vi "IntegrationNtimes.vi"(0 ".NET Refnum in":refnum<k24>, 1 "Port in":string, 2 "Array in":dbl[][](array[numeric]), 3 "ComError in":bool, 4 "tEnd":dbl, 5 "Burst # (M)":u32, 6 "error in":errorcluster, 7 "error in (no error)":errorcluster, 8 "VISA Refnum in":refnum<visa-resource-name>, 9 "Restart data point":bool, 10 "Array 2":i32[](array[numeric]), 11 "# of averages (N)":i64, 12 "Array 4":dbl[][](array[numeric]), 14 "Choose experiment":T1(ring), 16 "tEndCurrent":dbl) -> (17 "Numeric":i32, 18 "VISA resource name out":refnum<visa-resource-name>, 19 "ComError out 2":bool, 20 ".NET Refnum out":refnum<k24>, 21 "Numeric 2":dbl, 22 "Array":dbl[][](array[numeric]), 23 "Array out 2":dbl[][](array[numeric]), 24 "Array 3":dbl[][](array[numeric]), 25 "error out 3":errorcluster, 26 "Port out 2":string, 27 "error out":errorcluster)   [LabVIEW 2023]
uses:
  <vilib>/ULx/ULx_LV.dll
  <vilib>/ULx/Read.llb/ULx Read (Counter 1D U32 NChan 1Samp).vi
  <instrlib>/Quantum Composers 9000 Series/Quantum Composers 9000 Series.lvlib
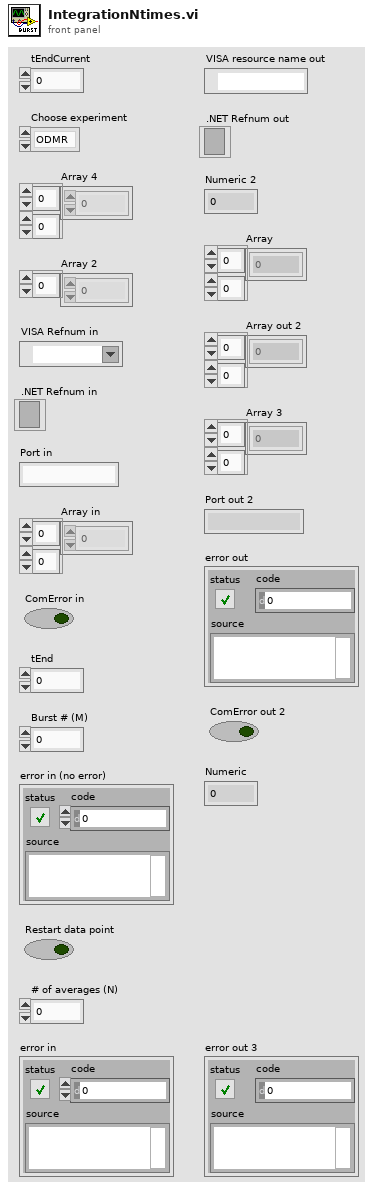
[diagram p1: front panel]
types:
  T1 = enum32{"ODMR", "Rabi", "Fidelity", "T1 Measurement"}
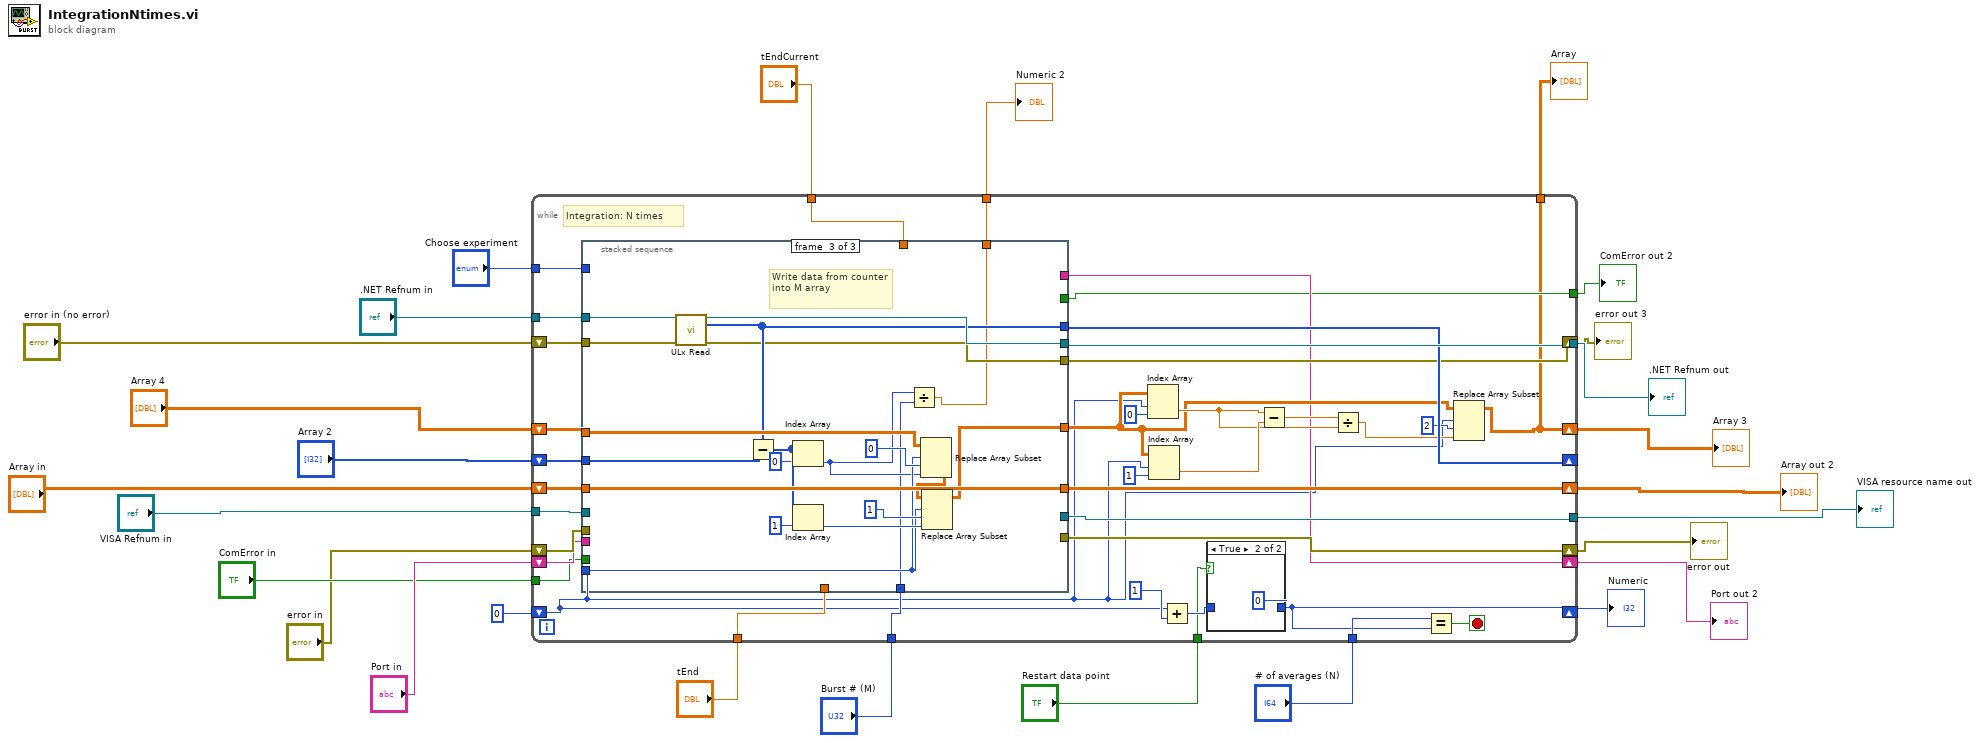
[diagram p0: block diagram]
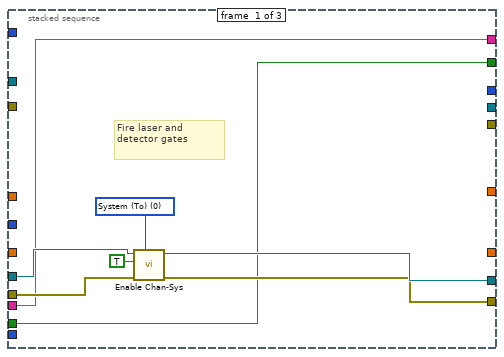
[diagram p2: hidden frame]
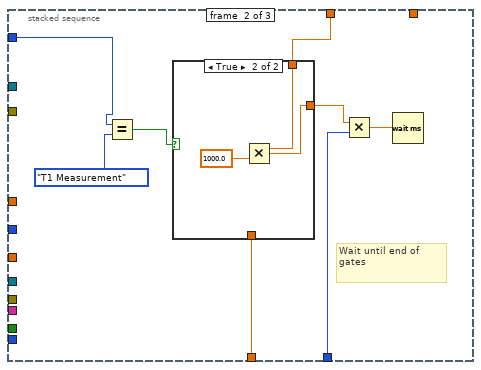
[diagram p3: hidden frame]
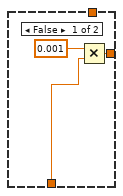
[diagram p4: hidden frame]
diagram:
  n1 = while {
    tunnel: [w65] -> w3
    tunnel: ".NET Refnum in" -> [w64]
    shift-right: [w62] -> w10
    shift-left: "Array in" -> [w61]
    shift-right: [w30] -> w7
    shift-left: "Array 4" -> [w60]
    shift-right: [w57] -> _
    shift-left: "Array 2" -> [w51]
    tunnel: [w43] -> w8
    shift-right: [w52] -> w1
    shift-left: "error in (no error)" -> [w63]
    shift-right: [w44] -> w11
    shift-left: "error in" -> [w53]
    tunnel: "VISA Refnum in" -> [w42]
    shift-right: [w40] -> w14
    shift-left: "Port in" -> [w41]
    tunnel: "ComError in" -> [w39]
    tunnel: [w38] -> w13
    tunnel: "tEndCurrent" -> [w37]
    tunnel: "Burst # (M)" -> [w36]
    tunnel: "tEnd" -> [w35]
    tunnel: "Choose experiment" -> [w34]
    tunnel: "# of averages (N)" -> [w33]
    tunnel: "Restart data point" -> [w32]
    tunnel: [w31] -> w25
    tunnel: [w30] -> w26
    shift-right: [w29] -> w27
    shift-left: 0 -> [w28]
    stop <- w54 stop-if-true
    # "Integration: N times"
    n2 = stacked-sequence {
      tunnel: w53 -> [w69 _ _]
      tunnel: w61 -> [_ _ w106]
      tunnel: [w71 _ _] -> w43
      tunnel: [_ _ w106] -> w62
      tunnel: [w70 _ _] -> w44
      tunnel: w64 -> [_ _ w104]
      tunnel: [_ _ w91] -> w52
      tunnel: [_ _ w107] -> w65
      tunnel: w63 -> [_ _ w105]
      tunnel: w28 -> [_ _ w93]
      tunnel: w60 -> [_ _ w98]
      tunnel: [_ _ w97] -> w47
      tunnel: w51 -> [_ _ w95]
      tunnel: [_ _ w96] -> w57
      tunnel: w42 -> [w68 _ _]
      tunnel: w41 -> [w67 _ _]
      tunnel: [w67 _ _] -> w40
      tunnel: w39 -> [w66 _ _]
      tunnel: [w66 _ _] -> w38
      tunnel: w37 -> [_ w77 _]
      tunnel: w36 -> [_ w76 w89]
      tunnel: w35 -> [_ w75 _]
      tunnel: w34 -> [_ w74 _]
      tunnel: [_ _ w88] -> w31
      frame #0 {
        w73 = 0 items=["System (To)", "Channel A", "Channel B", "Channel C", "Channel D", "Channel E", "Channel F", "Channel G", "Channel H"] ("Channel (1:Chan A)")
        # "Fire laser and detector gates"
        n3 = call <instrlib>:"Enable Chan-Sys.vi"("Channel (1:Chan A)"=w73, "error in (no error)"=w69, "State (T:Enabled)"=TRUE, "VISA resource name"=w68) -> ("error out"=w70:errorcluster, "VISA resource name out"=w71:refnum<visa-resource-name>)  [unwired: 6 in]
      }
      frame #1 {
        # "Wait until end of gates"
        n4 = Equal?(x=w74, y=T1."T1 Measurement") -> (x = y?=w79:bool)
        n5 = case shown="True" w79 {
          tunnel: [w83 w87] -> w81
          tunnel: w77 -> [_ w85]
          tunnel: w75 -> [w82 _]
          frame False {
            n6 = Multiply(x=0.001, y=w82) -> (x*y=w83:dbl)
          }
          frame True {
            n7 = Multiply(x=w85, y=1000.0) -> (x*y=w87:dbl)
          }
        }
        n8 = Multiply(x=w81, y=w76) -> (x*y=w80:dbl)
        n9 = Wait (ms)(milliseconds to wait=w80) -> ()  [unwired: 1 out]
      }
      frame #2 {
        # "Write data from counter into M array"
        n10 = call-poly <vilib>:"ULx Read.vi"("task in"=w104, "error in"=w105) -> ("task out"=w107:refnum<k24>, "data"=w96:u32[], "error out"=w91:errorcluster)  [unwired: 11 in]
        n11 = Subtract(x=w96, y=w95) -> (x-y=w103:u32[])
        n12 = Index Array(array=w103, index=0) -> (element=w92:u32)
        n13 = Index Array(array=w103, index=1) -> (element=w94:u32)
        n14 = Divide(x=w92, y=w89) -> (x/y=w88:dbl)
        n15 = Replace Array Subset(array=w98, new element=w92, index (row)=w93, index (col)=0) -> (w90:dbl[][])
        n16 = Replace Array Subset(array=w90, new element=w94, index (row)=w93, index (col)=1) -> (w97:dbl[][])
      }
    }
    n17 = Index Array(array=w47, index (row)=w28, index (col)=0 ("disabled index (col)")) -> (element=w48:dbl)
    n18 = Index Array(array=w47, index (row)=w28, index (col)=1 ("disabled index (col)")) -> (element=w50:dbl)
    n19 = Add(x=w28, y=1) -> (x+y=w55:i32)
    n20 = case shown="True" w32 {
      tunnel: [w108 0] -> w29
      tunnel: w55 -> [w108 _]
      frame False {
      }
      frame True {
      }
    }
    n21 = Subtract(x=w48, y=w50) -> (x-y=w49:dbl)
    n22 = Divide(x=w49, y=w48) -> (x/y=w45:dbl)
    n23 = Equal?(x=w33, y=w29) -> (x = y?=w54:bool)
    n24 = Replace Array Subset(array=w47, new element=w45, index (row)=w28, index (col)=2) -> (w30:dbl[][])
  }
  "Numeric" <- w27
  "Array" <- w26
  "Numeric 2" <- w25
  "Port out 2" <- w14
  "ComError out 2" <- w13
  "error out" <- w11
  "Array out 2" <- w10
  "error out 3" <- w1
  "VISA resource name out" <- w8
  "Array 3" <- w7
  ".NET Refnum out" <- w3
